vi "QMH Master Module Template.vi"   [LabVIEW 2018]
uses:
  Event Messaging/Type Defs/Event Message--cluster.ctl
  Event Messaging/Event Messaging.lvlib
  QMH Template/QMH Template.lvlib
types:
  T1 = typedef "Event Messaging.lvlib/Event Message--cluster.ctl" = cluster{"Cmd":string, "Data":variant}
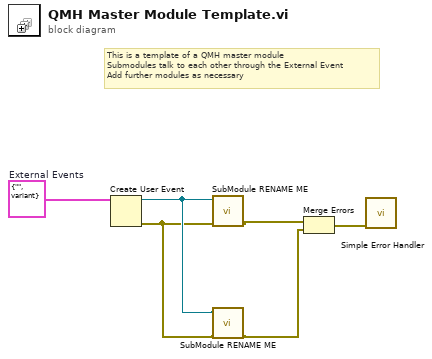
[diagram p0: block diagram]
diagram:
  w6 = T1 {"Cmd"="", "Data"=variant}  # External Events
  # "This is a template of a QMH master module\nSubmodules talk to each other through the External Event\nAdd further modules as necessary"
  n1 = Create User Event(user event datatype=w6) -> (user event=w3:refnum<user-event>, error out=w2:errorcluster)  [unwired: 1 in]
  n2 = call "SubModule RENAME ME.vi"("Error in"=w2, "External Event"=w3) -> ("Error out"=w4:errorcluster)  [unwired: 9 in]
  n3 = call "SubModule RENAME ME.vi"("Error in"=w2, "External Event"=w3) -> ("Error out"=w1:errorcluster)  [unwired: 9 in]
  n4 = Merge Errors(w4, w1) -> (w5:errorcluster)
  n5 = call <vilib>:"Simple Error Handler.vi"("error in (no error)"=w5) -> ()  [unwired: 4 in, 5 out]
